vi "PatientInfo.vi"(0 "refnum":refnum<file>, 9 "offset":i32) -> (2 "Patient Info":T2={"ID"="", "Extended ID"="", "age"=0, "gender"="", "previously\nscanned"="", "PSA"=0.0, "LOS"=1, "Ethnicty 3"=3, "Ethnicty 4"=3} {"Ethnicty 4" items=["Am Ind or Alaska", "Asian", "Hawaiian, Pac Isl", "Black or Afr Amer", "White", "more than one race", "unknown"]; "Ethnicty 3" items=["Hispanic", "Non-Hispanic", "unknown"]; "LOS" items=["1", "2", "3", "4", "5"]; "PSA" format="%.1f"}, 3 "blank":string, 4 "dup refnum":refnum<file>, 6 "ID":string, 8 "extended ID":string, 10 "age":u16, 11 "Ethnicity":u8, 12 "LOS":u8, 13 "PSA":sgl format="%.2f", 14 "previously scanned":string, 15 "sex":string)   [LabVIEW 2022 SP3]
panel:
  out "Patient Info Old":T1={"ID"="", "Extended ID"="", "age"=0, "gender"="", "previously\nscanned"="", "PSA"=0.0, "LOS"=1, "Ethnicty 3"=3} {"Ethnicty 3" items=["Am Ind or Alaska", "Asian, Pac Islander", "Black, not Hispanic", "Hispanic", "White, not hispanic", "other, unknown"]; "LOS" items=["1", "2", "3", "4", "5"]; "PSA" format="%.1f"}
  out "Race":u8(ring)=3 items=["Am Ind or Alaska", "Asian", "Hawaiian, Pac Isl", "Black or Afr Amer", "White", "more than one race", "unknown"]
  out "Ethnicty 1":u8(ring)=3 items=["Hispanic", "Non-Hispanic", "unknown"]
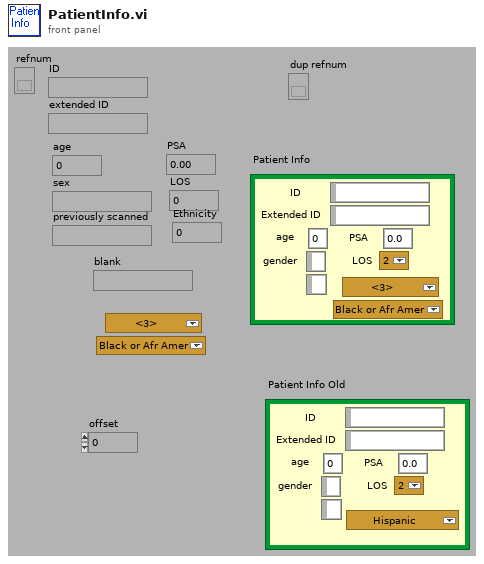
[diagram p1: front panel]
types:
  T1 = cluster{"ID":string, "Extended ID":string, "age":u16, "gender":string, "previously\nscanned":string, "PSA":sgl, "LOS":u8, "Ethnicty 3":u8}
  T2 = cluster{"ID":string, "Extended ID":string, "age":u16, "gender":string, "previously\nscanned":string, "PSA":sgl, "LOS":u8, "Ethnicty 3":u8, "Ethnicty 4":u8}
  T3 = cluster{string, string, u16, string, string, sgl, u8, i32, i32}
  T4 = cluster{string, string, u16, string, string, sgl, u8, u8}
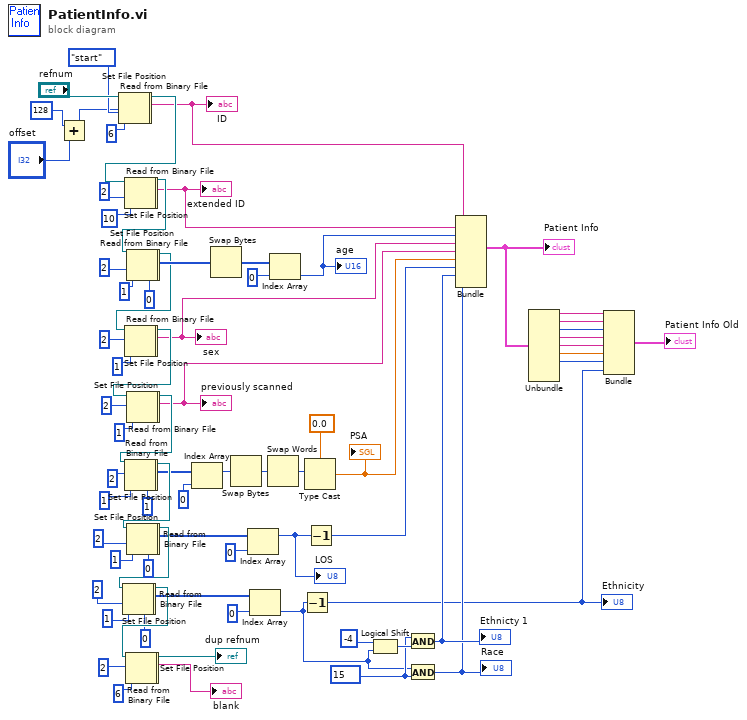
[diagram p0: block diagram]
diagram:
  w35 = 15
  n1 = Add(x=128 ("pos offset (0)"), y="offset") -> (x+y=w20:i32)
  n2 = Set File Position(offset (in bytes) (0)=w20, refnum="refnum", from (0:start)=enum16{"start", "end", "current"}."start" ("pos mode (0:2)")) -> (refnum out=w2:refnum<file>, error out=w1:errorcluster)  [unwired: 1 in]
  n3 = Read from Binary File(8:w1, 10:6 ("count"), 11:w2) -> (2:w68:string, 3:w86:refnum<file>)  [unwired: 5 out]
  "ID" <- w68
  n4 = Set File Position(refnum=w86, from (0:start)=2) -> (refnum out=w4:refnum<file>, error out=w3:errorcluster)  [unwired: 1 in, 1 out]
  n5 = Read from Binary File(8:w3, 10:10 ("count"), 11:w4) -> (2:w67:string, 3:w70:refnum<file>)  [unwired: 5 out]
  "extended ID" <- w67
  n6 = Set File Position(refnum=w70, from (0:start)=2) -> (refnum out=w12:refnum<file>, error out=w11:errorcluster)  [unwired: 1 in, 1 out]
  n7 = Read from Binary File(5:u16 0, 8:w11, 10:1 ("count"), 11:w12) -> (2:w77:u16[], 3:w73:refnum<file>)  [unwired: 4 out]
  n8 = Set File Position(refnum=w73, from (0:start)=2) -> (refnum out=w6:refnum<file>, error out=w5:errorcluster)  [unwired: 1 in, 1 out]
  n9 = Read from Binary File(8:w5, 10:1 ("count"), 11:w6) -> (2:w66:string, 3:w72:refnum<file>)  [unwired: 5 out]
  "sex" <- w66
  n10 = Set File Position(refnum=w72, from (0:start)=2) -> (refnum out=w8:refnum<file>, error out=w7:errorcluster)  [unwired: 1 in, 1 out]
  n11 = Read from Binary File(8:w7, 10:1 ("count"), 11:w8) -> (2:w63:string, 3:w71:refnum<file>)  [unwired: 5 out]
  "previously scanned" <- w63
  n12 = Set File Position(refnum=w71, from (0:start)=2) -> (refnum out=w14:refnum<file>, error out=w13:errorcluster)  [unwired: 1 in, 1 out]
  n13 = Read from Binary File(5:1 ("count"), 8:w13, 10:1 ("count"), 11:w14) -> (2:w40:i32[], 3:w58:refnum<file>)  [unwired: 4 out]
  n14 = Set File Position(refnum=w58, from (0:start)=2) -> (refnum out=w16:refnum<file>, error out=w15:errorcluster)  [unwired: 1 in, 1 out]
  n15 = Read from Binary File(5:u8 0, 8:w15, 10:1 ("count"), 11:w16) -> (2:w44:u8[], 3:w57:refnum<file>)  [unwired: 4 out]
  n16 = Set File Position(refnum=w57, from (0:start)=2) -> (refnum out=w18:refnum<file>, error out=w17:errorcluster)  [unwired: 1 in, 1 out]
  n17 = Read from Binary File(5:u8 0, 8:w17, 10:1 ("count"), 11:w18) -> (2:w41:u8[], 3:w56:refnum<file>)  [unwired: 4 out]
  n18 = Set File Position(refnum=w56, from (0:start)=2) -> (refnum out=w10:refnum<file>, error out=w9:errorcluster)  [unwired: 1 in, 1 out]
  n19 = Read from Binary File(8:w9, 10:6 ("count"), 11:w10) -> (2:→"blank":string, 3:→"dup refnum":refnum<file>)  [unwired: 5 out]
  n20 = Index Array(array=w40, index=0) -> (element=w39:i32)
  n21 = Swap Bytes(anything=w77) -> (byte swapped=w65:u16[])
  n22 = Swap Bytes(anything=w39) -> (byte swapped=w53:i32)
  n23 = Index Array(array=w44, index=0) -> (element=w43:u8)
  "LOS" <- w43
  n24 = Index Array(array=w41, index=0) -> (element=w34:u8)
  n25 = Swap Words(1:w53) -> (0:w52:i32)
  n26 = Index Array(array=w65, index=0) -> (element=w64:u16)
  "age" <- w64
  n27 = Decrement(x=w34) -> (x-1=w23:u8)
  "Ethnicity" <- w23
  n28 = Type Cast(type=sgl 0.0, x=w52) -> (*(type *) &x=w49:sgl)
  "PSA" <- w49
  n29 = Decrement(x=w43) -> (x-1=w48:u8)
  n30 = Logical Shift(y=-4, x=w34) -> (x << y=w36:u8)
  n31 = And(x=w35, y=w36) -> (x .and. y?=w33:i32)
  "Ethnicty 1" <- w33
  n32 = And(x=w34, y=w35) -> (x .and. y?=w32:i32)
  "Race" <- w32
  n33 = Bundle(w68, w67, w64, w66, w63, w49, w48, w33, w32) -> (w31:T3)  [unwired: 1 out]
  "Patient Info" <- w31
  n34 = Unbundle(w31) -> (w30:string, w29:string, w28:u16, w27:string, w26:string, w25:sgl, w24:u8)  [unwired: 2 out]
  n35 = Bundle(w30, w29, w28, w27, w26, w25, w24, w23) -> (→"Patient Info Old":T4)  [unwired: 1 out]
